vi "Parametric Sweep - Environment.vi"() -> ()   [LabVIEW 2013]
uses:
  DMM/Signal Types.ctl
  Power Supply.lvlib
  Fixture.lvlib
  DMM.lvlib
panel:
  in  "Resolution":i32=10
  in  "serial number":string="1"
  out "Intensity Graph":dbl[][](graph)
  in  "Channel":i32=6
  out "error out":errorcluster
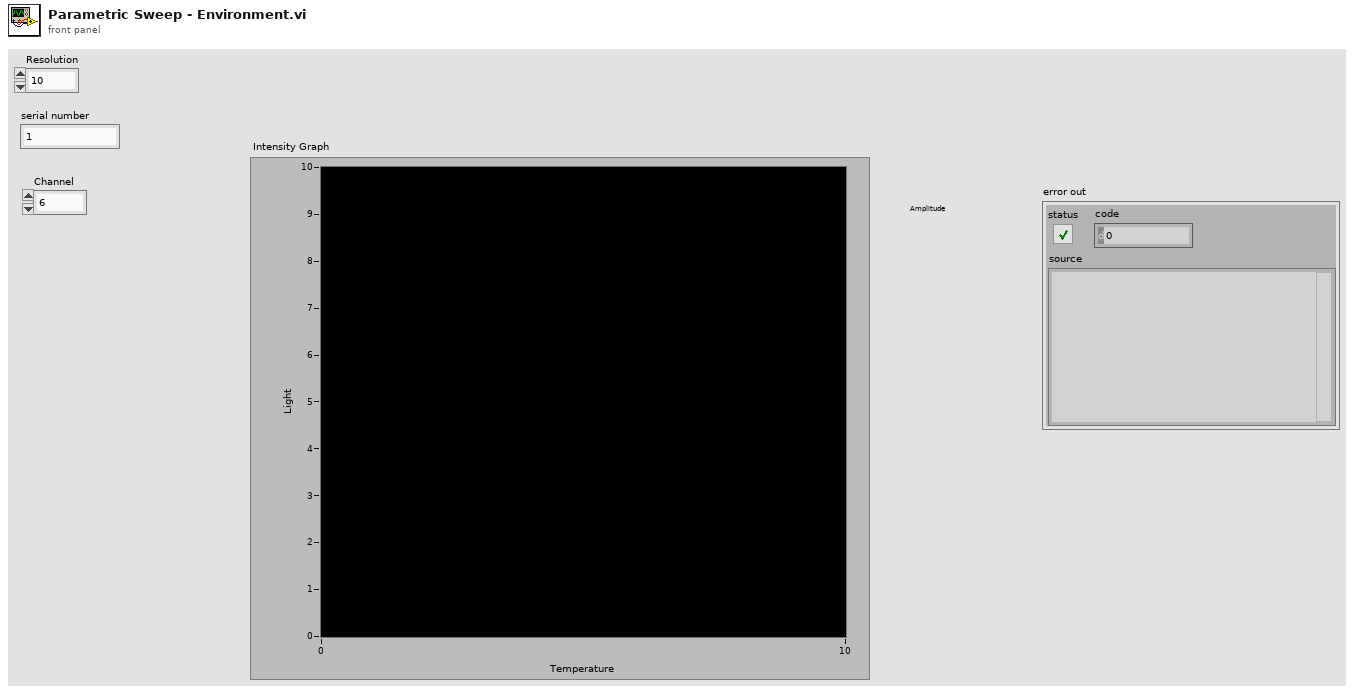
[diagram p1: front panel]
types:
  T1 = typedef "Driver Simulation.lvlib/DMM.lvlib/Signal Types.ctl" = enum16{"DC", "AC"}
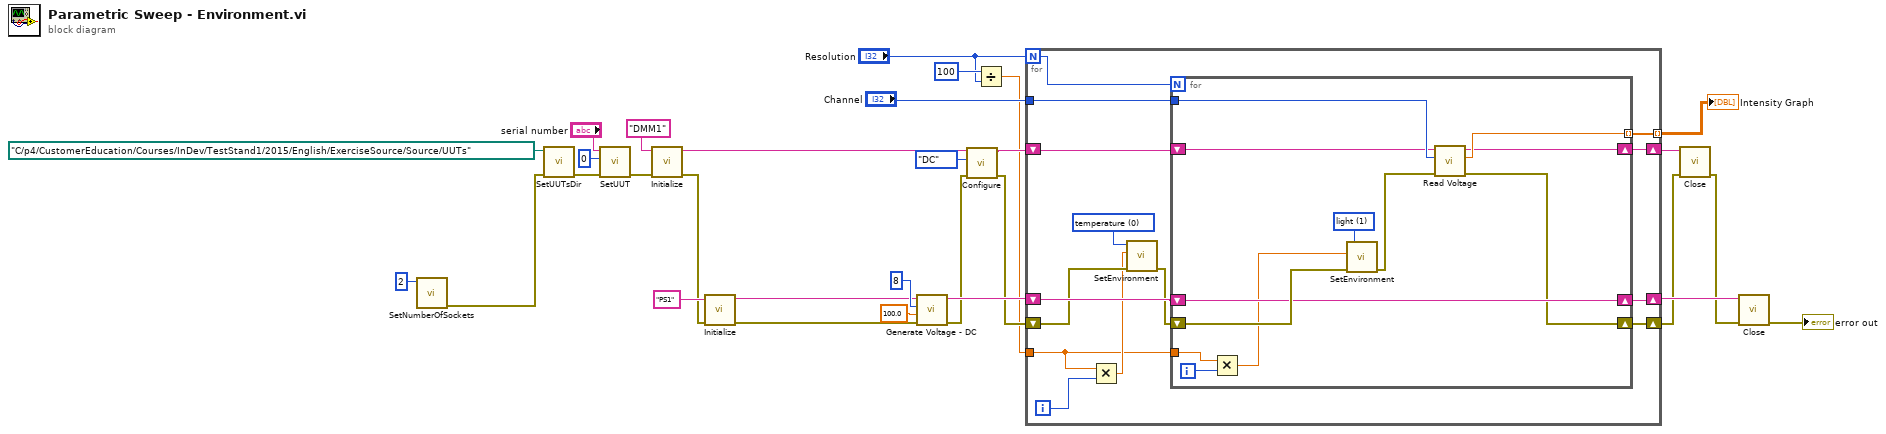
[diagram p0: block diagram]
diagram:
  n1 = call "SetNumberOfSockets.vi"("Number of Sockets"=2) -> ("error out"=w5:errorcluster)  [unwired: 10 in]
  n2 = call "SetUUTsDir.vi"("error in (no error)"=w5, "UUTDirectory"=path "C:/p4/CustomerEducation/Courses/InDev/TestStand1/2015/English/ExerciseSource/Source/UUTs") -> ("error out"=w30:errorcluster)  [unwired: 9 in]
  n3 = call "SetUUT.vi"("error in (no error)"=w30, "Test Socket (0)"=0 ("socketIndex (0)"), "Serial Number"="serial number") -> ("error out"=w17:errorcluster)  [unwired: 8 in]
  n4 = call "Initialize.vi"("error in (no error)"=w17, "DMM in"="DMM1" ("Resource Name")) -> ("error out"=w16:errorcluster, "DMM out"=w15:string)  [unwired: 8 in]
  n5 = call "Initialize.vi"("error in (no error)"=w16, "Power Supply in"="PS1" ("Resource Name")) -> ("error out"=w1:errorcluster, "Power Supply out"=w2:string)  [unwired: 8 in]
  n6 = call "Generate Voltage - DC.vi"("error in (no error)"=w1, "Output Voltage"=100.0 ("outputVoltage"), "Channel"=8 ("channel"), "Power Supply in"=w2) -> ("error out"=w14:errorcluster, "Power Supply out"=w20:string)  [unwired: 6 in]
  n7 = call "Configure.vi"("error in (no error)"=w14, "Signal Type"=Signal_Types."DC" ("signalType"), "DMM in"=w15) -> ("error out"=w13:errorcluster, "DMM out"=w19:string)  [unwired: 7 in]
  n8 = Divide(x=100, y="Resolution") -> (x/y=w6:dbl)
  n9 = for {
    N: "Resolution" -> [w36]
    tunnel: "Channel" -> [w40]
    tunnel: [w39] -> w23 mode=indexing
    shift-right: [w44] -> w12
    shift-left: w13 -> [w35]
    tunnel: w6 -> [w32]
    shift-right: [w43] -> w10
    shift-left: w19 -> [w42]
    shift-right: [w41] -> w29
    shift-left: w20 -> [w38]
    i -> [w34]
    w31 = 0 items=["temperature", "light"] ("setting")
    n10 = Multiply(x=w32, y=w34) -> (x*y=w33:dbl)
    n11 = call "SetEnvironment.vi"("error in (no error)"=w35, "Value"=w33, "Setting"=w31) -> ("error out"=w37:errorcluster)  [unwired: 8 in]
    n12 = for {
      N: w36 -> [_]
      tunnel: w40 -> [w51]
      shift-right: [w55] -> w41
      shift-left: w38 -> [w55]
      shift-right: [w49] -> w43
      shift-left: w42 -> [w50]
      tunnel: [w52] -> w39 mode=indexing
      shift-right: [w53] -> w44
      shift-left: w37 -> [w56]
      tunnel: w32 -> [w48]
      i -> [w47]
      w45 = 1 items=["temperature", "light"] ("setting")
      n13 = Multiply(x=w48, y=w47) -> (x*y=w46:dbl)
      n14 = call "SetEnvironment.vi"("error in (no error)"=w56, "Value"=w46, "Setting"=w45) -> ("error out"=w54:errorcluster)  [unwired: 8 in]
      n15 = call "Read Voltage.vi"("error in (no error)"=w54, "Channel"=w51, "DMM in"=w50) -> ("error out"=w53:errorcluster, "Voltage"=w52:dbl, "DMM out"=w49:string)  [unwired: 6 in]
    }
  }
  "Intensity Graph" <- w23
  n16 = call "Close.vi"("error in (no error)"=w12, "DMM in"=w10) -> ("error out"=w11:errorcluster)  [unwired: 9 in]
  n17 = call "Close.vi"("error in (no error)"=w11, "Power Supply in"=w29) -> ("error out"=→"error out":errorcluster)  [unwired: 9 in]
